vi "ziSetValueInt.vi"(3 "Error in":errorcluster, 4 "Value":i64, 5 "Path":string, 6 "Handle in":T1 {"Handle" format="0x%08x"; "Conn" format="0x%08x"}) -> (0 "Error out":errorcluster, 2 "Handle out":T1 {"Handle" format="0x%08x"; "Conn" format="0x%08x"})   [LabVIEW 2009, in "Zurich Instruments LabOne.lvlib"]
doc: "---Obsolete---"
uses:
  <instrlib>/Zurich Instruments LabOne/Zurich Instruments LabOne.lvlib
  <instrlib>/Zurich Instruments LabOne/Public/ziTypeHandle.ctl
  <instrlib>/Zurich Instruments LabOne/Private/ziLV32.dll
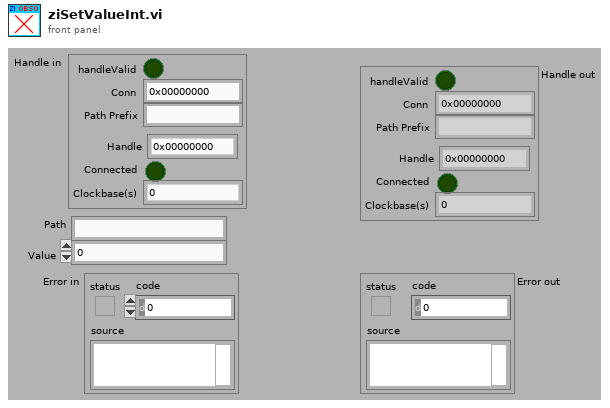
[diagram p1: front panel]
types:
  T1 = typedef "Zurich Instruments LabOne.lvlib/ziTypeHandle.ctl" = cluster{"handleValid":bool, "Conn":u64, "Path Prefix":string, "Handle":u64, "Connected":bool, "Clockbase(s)":dbl}
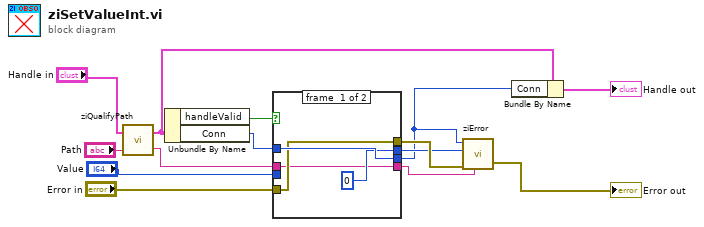
[diagram p0: block diagram]
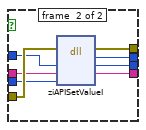
[diagram p2: hidden frame]
diagram:
  n1 = call <instrlib>:"ziQualifyPath.vi"("Path In"="Path", "Handle In"="Handle in") -> ("Path Out"=w2:string, "Handle Out"=w3:T1)
  n2 = Unbundle By Name(w3) -> ("handleValid"=w8:bool, "Conn"=w13:u64)
  n3 = case shown="True" w8 {
    tunnel: "Error in" -> [w17 w26]
    tunnel: w13 -> [w18 w25]
    tunnel: w2 -> [w15 w24]
    tunnel: "Value" -> [_ w23]
    tunnel: [w17 w22] -> w10
    tunnel: [u32 0 ("return type") w21] -> w9
    tunnel: [w18 w20] -> w1
    tunnel: [w15 w19] -> w6
    frame #0 {
    }
    frame #1 {
      n4 = dll-call lib="C:/Program Files (x86)/National Instruments/LabVIEW 2009/instr.lib/Zurich Instruments LabOne/Private/ziLV*.*" fn="ziAPISetValueI"(error in=w26, "Conn"=w25, "Path"=w24, "Value"=w23) -> (error out=w22:errorcluster, "return type"=w21:u32, "Conn"=w20:u64, "Path"=w19:string)  [unwired: 3 in, 1 out]
    }
  }
  n5 = call <instrlib>:"ziError.vi"("Conn"=w1, "ziErrorCode"=w9, "Error In"=w10, "Annotation"=w6) -> ("Error Out"=→"Error out":errorcluster)  [unwired: 1 in, 1 out]
  n6 = Bundle By Name(cluster=w3, "Conn"=w1) -> (→"Handle out":T1)
